vi "matrici_v0_v38.vi"() -> ()   [LabVIEW 2009]
panel:
  in  "stop":bool
  in  "Slide":u8(slide) scale=0.0..9.0
  out "Array 2":bool[][](array[boolean])
  in  "Array":bool[][][](array[boolean])
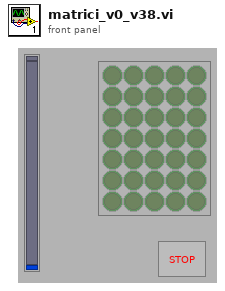
[diagram p1: front panel]
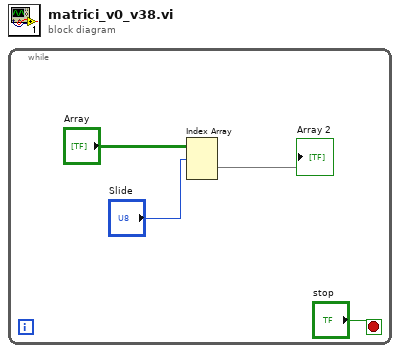
[diagram p0: block diagram]
diagram:
  n1 = while {
    stop <- "stop" stop-if-true
    n2 = Index Array(array="Array", index (dim 0)="Slide") -> (element=→"Array 2":bool[][])  [unwired: 2 in]
  }
